vi "Serial reader.vi"() -> ()   [LabVIEW 2018]
uses:
  Configuration.lvlib
panel:
  out "error out":errorcluster
  in  "error in (no error)":errorcluster
  out "String":string
  in  "Keys":string[](array[string])=["Resource Name", "Baud Rate", "Data Bits", "Parity"]
  in  "Section":string
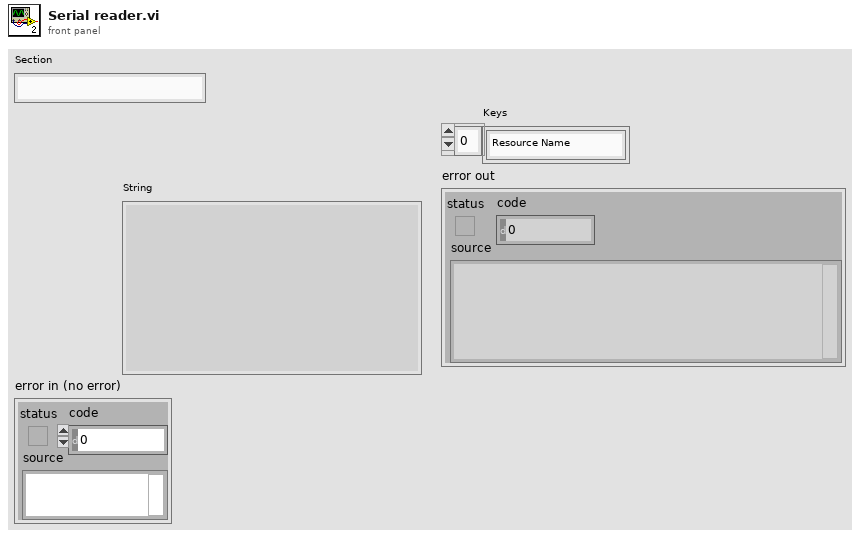
[diagram p1: front panel]
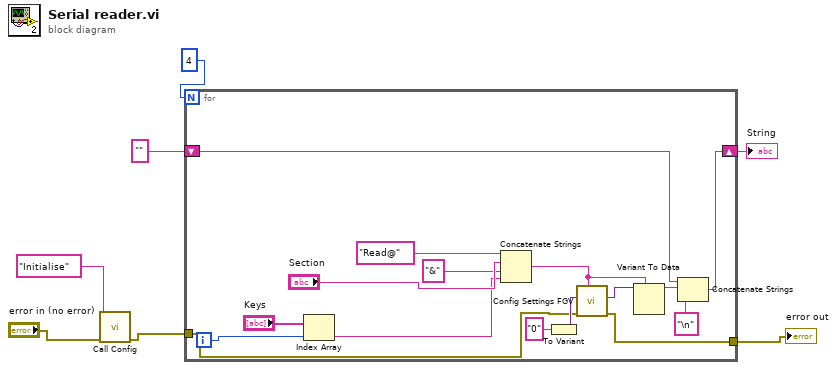
[diagram p0: block diagram]
diagram:
  n1 = call "Call Config.vi"("error in (no error)"="error in (no error)", "Command"="Initialise") -> ("error out"=w1:errorcluster)  [unwired: 9 in]
  n2 = for {
    N: 4 -> [_]
    shift-right: [w11] -> w5
    shift-left: "" -> [w8]
    tunnel: [w10] -> w4
    tunnel: w1 -> [w9]
    i -> [w19]
    n3 = Index Array(array="Keys", index=w19) -> (element=w18:string)
    n4 = Concatenate Strings("Read@", "Section", "&", w18) -> (w15:string)
    n5 = To Variant(anything="0") -> (Variant=w16:variant)
    n6 = call "Config Settings FGV.vi"("Command"=w15, "error in (no error)"=w9, "Data in"=w16) -> ("error out"=w10:errorcluster, "Data out"=w14:variant)  [unwired: 7 in]
    n7 = Variant To Data(type=w15, Variant=w14) -> (data=w13:string)  [unwired: 1 in, 1 out]
    n8 = Concatenate Strings(w8, w13, "\n" ("string")) -> (w11:string)
  }
  "String" <- w5
  "error out" <- w4
